vi "Host_PhotonCounter.vi"() -> ()   [LabVIEW 2012]
uses:
  <vilib>/FPGAPlugInAG/PXIe-7962R/niLvFpga_Open_PXIe-7962R.vi
  <vilib>/rvi/interface/common/dynamic/niFpgaDynamicAddResources.vi
  <vilib>/FPGAPlugInAG/Dynamic/niLvFpga_Reset_Dynamic.vi
  <vilib>/Utility/error.llb/Error Cluster From Error Code.vi
  <vilib>/rvi/errors/niLvFpgaAdjustHostInterfaceError.vi
  <vilib>/FPGAPlugInAG/Dynamic/niLvFpga_Close_Dynamic.vi
  <vilib>/rvi/interface/nirviOpenFPGA/nirviOpenFPGA.xnode
  FPGA Bitfiles/PhotonCounterV2_PXIe-7962R.lvbitx
  <vilib>/rvi/interface/nirviMethod/nirviMethod.xnode
  <vilib>/rvi/interface/nirviReadWriteControl/nirviReadWriteControl.xnode
  <vilib>/rvi/interface/nirviCloseFPGA/nirviCloseFPGA.xnode
  <vilib>/rvi/interface/Simulation/niFpgaSimulationCallBeginRW.vi
  NiFpgaLv.dll
  <vilib>/FPGAPlugInAG/Dynamic/niLvFpga_ReadFifo_Dynamic.vi
  <vilib>/rvi/errors/niLvFpgaMergeErrorWithErrorCode.vi
panel:
  out "Elements Remaining Ch2":u32
  out "Elements Remaining Ch1":u32
  out "Ch2:0":u16
  out "Ch1:0":u16
  out "Acquiring":bool
  out "ToHost FIFO Overflow Ch2":bool
  out "ToHost FIFO Overflow Ch1":bool
  out "Laser pulses per pixel":dbl
  in  "Laser pulse frequency":dbl=80000000.0 format="%#_6p"
  in  "Samples per pixel":u16=10000
  out "Pixel time":dbl
  out "Acquired samples":u32
  out "Interloop FIFO overflow":bool
  out "Interloop FIFO timeout":bool
  in  "Reset":bool
  in  "Quit":bool
  out "Sampling frequency":dbl format="%#_6p"
  out "Sampling interval":dbl format="%#_6p"
  in  "Onboard clock frequency":dbl=500000000.0 format="%#_6p"
  # "Configuration"
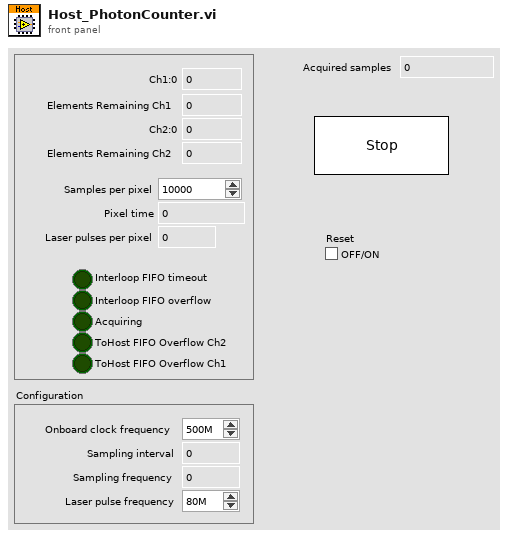
[diagram p1: front panel]
types:
  T1 = enum8{"Enabled", "Disabled", "Disabled and Grayed Out"}
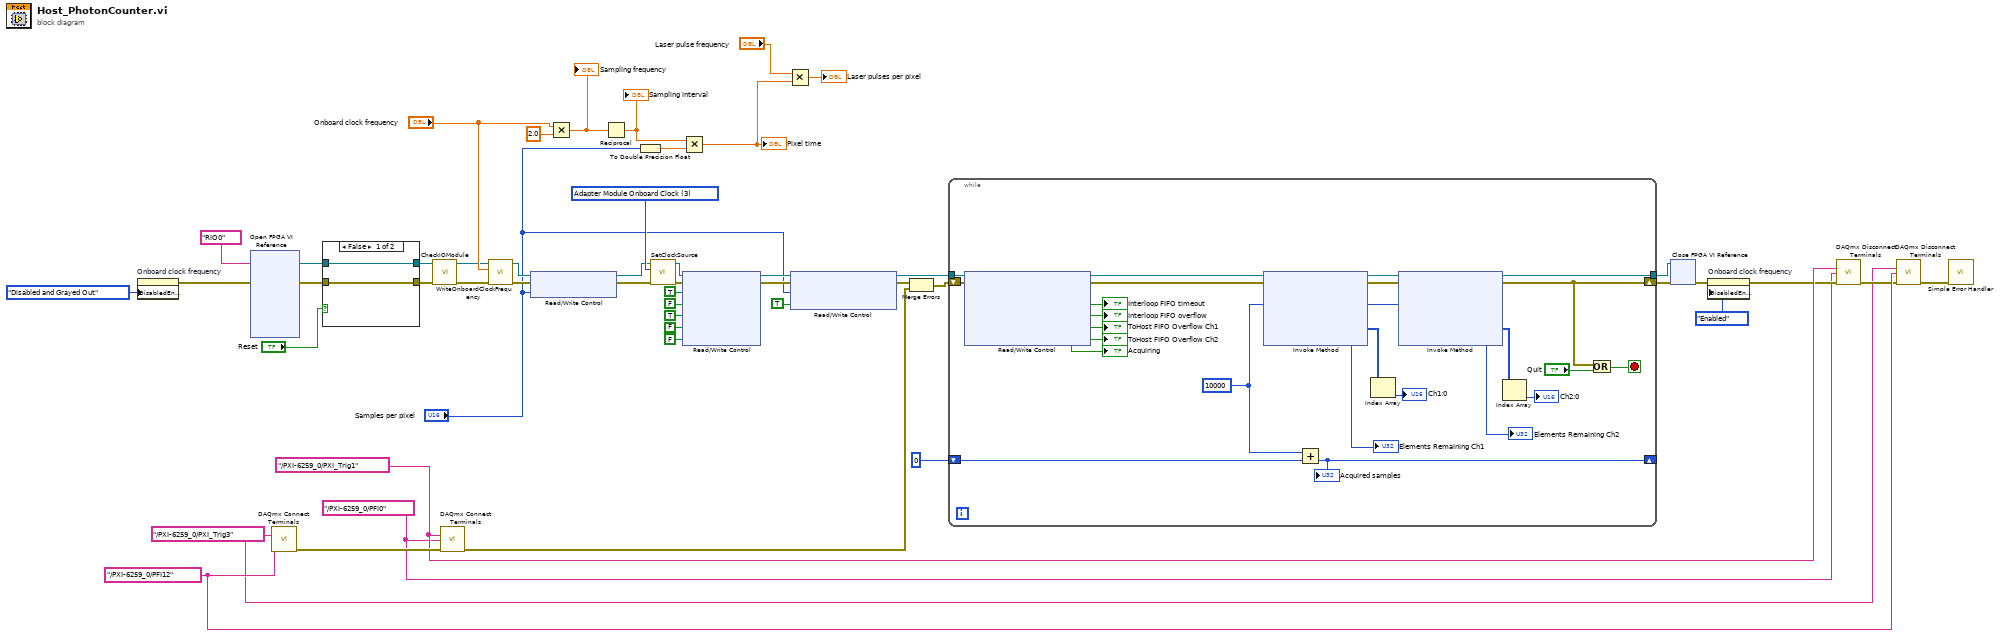
[diagram p0: block diagram]
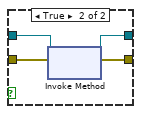
[diagram p2: hidden frame]
diagram:
  w9 = tag "/PXI-6259_0/PFI0" ("destination terminal")
  w14 = tag "/PXI-6259_0/PXI_Trig1" ("source terminal")
  w17 = tag "/PXI-6259_0/PFI12" ("destination terminal")
  w10 = tag "/PXI-6259_0/PXI_Trig3" ("source terminal")
  w51 = u8 3 items=["Tristate"=0, "Sync Clock (PXIe only)"=2, "Adapter Module Onboard Clock"=3, "Strobe from Crosspoint Switch"=4, "Strobe Bypass"=5] ("Clock Source")
  n1 = property on="Onboard clock frequency" class="DigNum (strict)"("DisabledEnum"=T1."Disabled and Grayed Out" ("Disabled")) -> (error out=w40:errorcluster)  [unwired: 2 in, 1 out]
  n2 = xnode "Open FPGA VI Reference"("error in"=w40, "resource name"=tag "RIO0") -> ("FPGA VI Reference Out"=w27:refnum<k20>, "error out"=w25:errorcluster)
  n3 = call <vilib>:"DAQmx Connect Terminals.vi"("source terminal"=w10, "destination terminal"=w17) -> ("error out"=w16:errorcluster)  [unwired: 13 in]
  n4 = case shown="False" "Reset" {
    tunnel: w27 -> [w52 w57]
    tunnel: [w52 w56] -> w26
    tunnel: w25 -> [w53 w55]
    tunnel: [w53 w54] -> w24
    frame False {
    }
    frame True {
      n5 = xnode "Invoke Method"("FPGA VI Reference In"=w57, "error in"=w55) -> ("FPGA VI Reference Out"=w56:refnum<k20>, "error out"=w54:errorcluster)
    }
  }
  n6 = call "CheckIOModule.vi"("error in (no error)"=w24, "FPGA VI Reference In"=w26) -> ("error out"=w44:errorcluster, "FPGA VI Reference Out"=w36:refnum<k20>)  [unwired: 8 in]
  n7 = call <vilib>:"DAQmx Connect Terminals.vi"("source terminal"=w14, "destination terminal"=w9, "error in"=w16) -> ("error out"=w15:errorcluster)  [unwired: 12 in]
  n8 = call "WriteOnboardClockFrequency.vi"("error in (no error)"=w44, "Onboard clock frequency"="Onboard clock frequency", "FPGA VI Reference In"=w36) -> ("error out"=w35:errorcluster, "FPGA VI Reference Out"=w33:refnum<k20>)  [unwired: 7 in]
  n9 = xnode "Read/Write Control"("FPGA VI Reference In"=w33, "error in"=w35, "Samples per pixel"="Samples per pixel") -> ("FPGA VI Reference Out"=w32:refnum<k20>, "error out"=w34:errorcluster)
  n10 = Multiply(x="Onboard clock frequency", y=2.0) -> (x*y=w41:dbl)
  "Sampling frequency" <- w41
  n11 = Reciprocal(x=w41) -> (1/x=w30:dbl)
  "Sampling interval" <- w30
  n12 = To Double Precision Float(number="Samples per pixel") -> (double precision float=w29:dbl)
  n13 = call "SetClockSource.vi"("error in (no error)"=w34, "Clock Source"=w51, "FPGA VI Reference In"=w32) -> ("error out"=w49:errorcluster, "FPGA VI Reference Out"=w50:refnum<k20>)  [unwired: 7 in]
  n14 = Multiply(x=w30, y=w29) -> (x*y=w20:dbl)
  "Pixel time" <- w20
  n15 = xnode "Read/Write Control"("FPGA VI Reference In"=w50, "error in"=w49, "Commit"=TRUE, "Acq_Reset"=FALSE, "Acq_Reset"=TRUE, "Acq_Reset"=FALSE, "Wait for trigger"=FALSE) -> ("FPGA VI Reference Out"=w7:refnum<k20>, "error out"=w8:errorcluster)
  n16 = Multiply(x="Laser pulse frequency", y=w20) -> (x*y=→"Laser pulses per pixel":dbl)
  n17 = xnode "Read/Write Control"("FPGA VI Reference In"=w7, "error in"=w8, "Samples per pixel Acq"="Samples per pixel", "Acquire"=TRUE) -> ("FPGA VI Reference Out"=w5:refnum<k20>, "error out"=w6:errorcluster)
  n18 = Merge Errors(w6, w15) -> (w18:errorcluster)
  n19 = while {
    shift-right: [w66] -> w31
    shift-left: w18 -> [w79]
    shift-right: [w75] -> _
    shift-left: u32 0 -> [w76]
    tunnel: w5 -> [w74]
    tunnel: [w65] -> w2
    stop <- w80 stop-if-true
    w64 = u32 10000 ("Number of Elements")
    n20 = xnode "Read/Write Control"("FPGA VI Reference In"=w74, "error in"=w79) -> ("FPGA VI Reference Out"=w69:refnum<k20>, "error out"=w70:errorcluster, "Interloop FIFO timeout"=→"Interloop FIFO timeout":bool, "Interloop FIFO overflow"=→"Interloop FIFO overflow":bool, "ToHost FIFO Overflow Ch1"=→"ToHost FIFO Overflow Ch1":bool, "ToHost FIFO Overflow Ch2"=→"ToHost FIFO Overflow Ch2":bool, "Acquiring"=→"Acquiring":bool)
    n21 = xnode "Invoke Method"("FPGA VI Reference In"=w69, "error in"=w70, "Number of Elements"=w64) -> ("FPGA VI Reference Out"=w68:refnum<k20>, "error out"=w67:errorcluster, "Data"=w63:u16[], "Elements Remaining"=→"Elements Remaining Ch1":u32)  [unwired: 1 in]
    n22 = Add(x=w64, y=w76) -> (x+y=w75:u32)
    "Acquired samples" <- w75
    n23 = Index Array(array=w63) -> (element=→"Ch1:0":u16)  [unwired: 1 in]
    n24 = xnode "Invoke Method"("FPGA VI Reference In"=w68, "error in"=w67, "Number of Elements"=w64) -> ("FPGA VI Reference Out"=w65:refnum<k20>, "error out"=w66:errorcluster, "Data"=w62:u16[], "Elements Remaining"=→"Elements Remaining Ch2":u32)  [unwired: 1 in]
    n25 = Index Array(array=w62) -> (element=→"Ch2:0":u16)  [unwired: 1 in]
    n26 = Or(x=w66, y="Quit") -> (x .or. y?=w80:bool)
  }
  n27 = xnode "Close FPGA VI Reference"("FPGA VI Reference In"=w2, "error in"=w31) -> ("error out"=w38:errorcluster)
  n28 = property on="Onboard clock frequency" class="DigNum (strict)"(error in=w38, "DisabledEnum"=T1."Enabled" ("Disabled")) -> (error out=w13:errorcluster)  [unwired: 1 in, 1 out]
  n29 = call <vilib>:"DAQmx Disconnect Terminals.vi"("source terminal"=w14, "destination terminal"=w9, "error in"=w13) -> ("error out"=w12:errorcluster)  [unwired: 12 in]
  n30 = call <vilib>:"DAQmx Disconnect Terminals.vi"("source terminal"=w10, "destination terminal"=w17, "error in"=w12) -> ("error out"=w11:errorcluster)  [unwired: 12 in]
  n31 = call <vilib>:"Simple Error Handler.vi"("error in (no error)"=w11) -> ()  [unwired: 4 in, 5 out]
